vi "FGV - Path Registration.vi"(7 "FGV State":T1=enum."Register Path", 8 "error in (no error)":errorcluster, 10 "Path":path, 11 "Key":variant) -> (0 "error out":errorcluster, 1 "Key Already Included?":bool, 2 "Key Not Found?":bool, 3 "Path Out":path, 4 "Value Unchanged?":bool, 5 "All Paths":path[](array[path]))   [LabVIEW 2021, in "Path Utilities.lvlib"]
doc: "FGV for \"Path Registration\" VIs.\nNo error are generated inside this FGV."
uses:
  Path Utilities.lvlib
  TypeDefs/FGV State - Path Registration.ctl
  TypeDefs/FGV Data - Path Registration.ctl
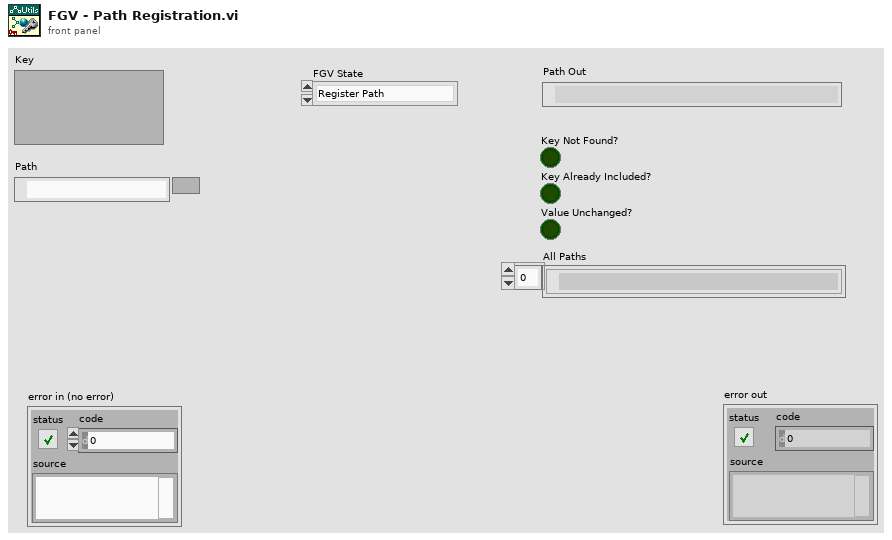
[diagram p1: front panel]
types:
  T1 = typedef "Path Utilities.lvlib/FGV State - Path Registration.ctl" = enum16{"Get Path", "List All Paths", "Register Path", "Unregister Path"}
  T2 = typedef "Path Utilities.lvlib/FGV Data - Path Registration.ctl" = cluster{"Path Map":map{variant, path}}
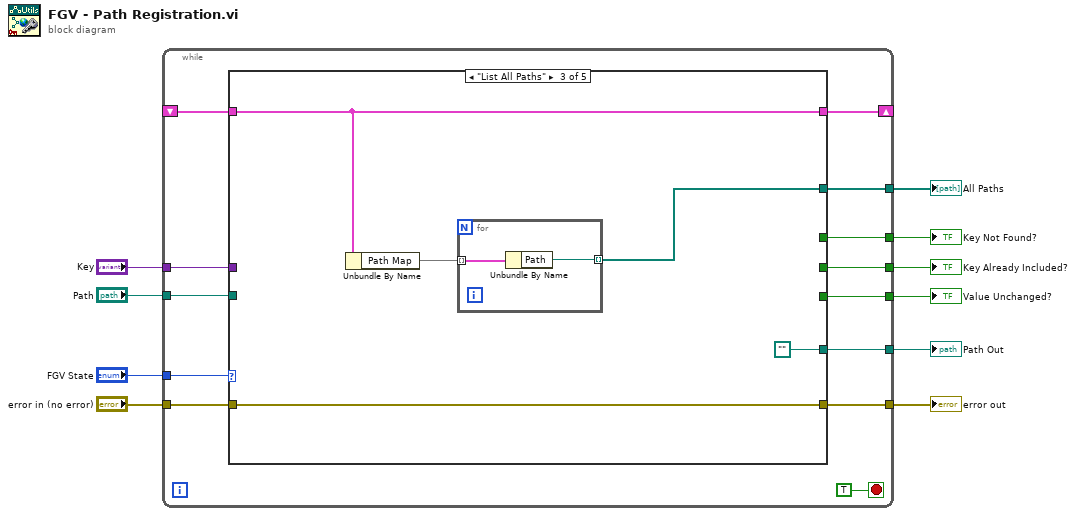
[diagram p0: block diagram]
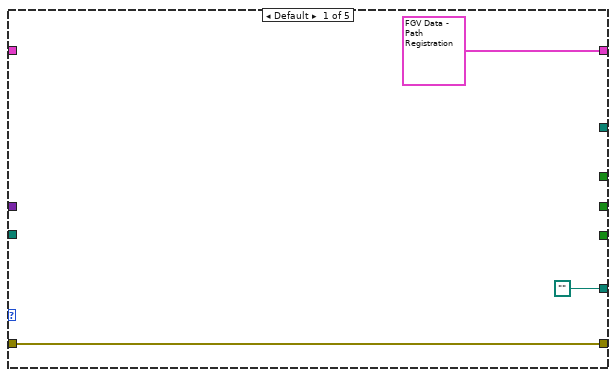
[diagram p2: hidden frame]
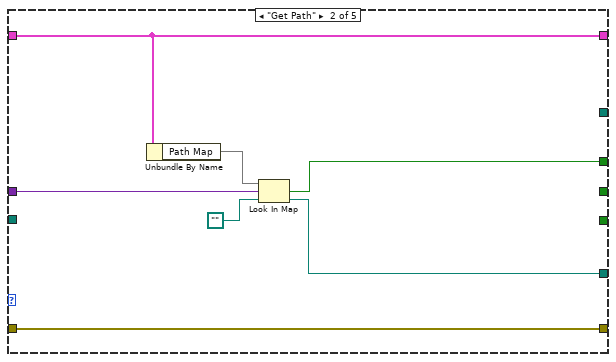
[diagram p3: hidden frame]
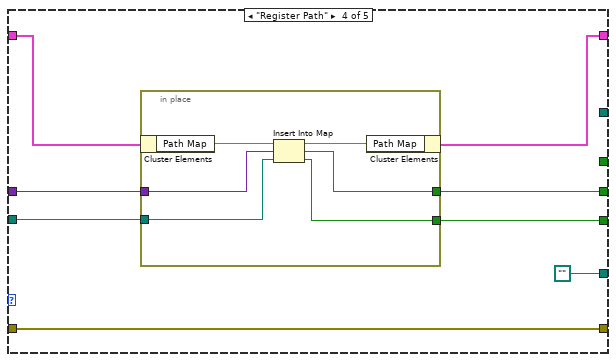
[diagram p4: hidden frame]
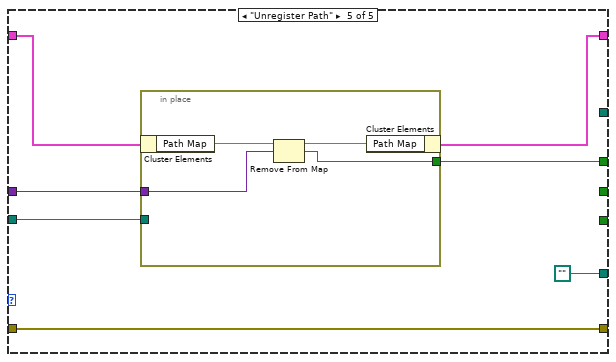
[diagram p5: hidden frame]
diagram:
  n1 = while {
    shift-right: [w19] -> _
    shift-left: _ -> [w17]
    tunnel: "FGV State" -> [w22]
    tunnel: "error in (no error)" -> [w21]
    tunnel: [w20] -> w9
    tunnel: "Path" -> [w18]
    tunnel: "Key" -> [w16]
    tunnel: [w15] -> w5
    tunnel: [w14] -> w4
    tunnel: [w13] -> w3
    tunnel: [w12] -> w2
    tunnel: [w11] -> w1
    stop <- TRUE stop-if-true
    n2 = case shown="\"List All Paths\"" w22 {
      tunnel: w21 -> [w26 w27 w35 w44 w57]
      tunnel: [w26 w27 w35 w44 w57] -> w20
      tunnel: [T2 {"Path Map"={}} ("FGV Data") w33 w38 w47 w60] -> w19
      tunnel: w18 -> [_ _ _ w45 w58]
      tunnel: w17 -> [_ w33 w38 w48 w61]
      tunnel: w16 -> [_ w32 _ w46 w59]
      tunnel: [_ _ _ w43 _] -> w15
      tunnel: [_ _ _ w42 _] -> w14
      tunnel: [path "" w29 path "" path "" path ""] -> w13
      tunnel: [_ w28 _ _ w56] -> w12
      tunnel: [_ _ w36 _ _] -> w11
      frame Default {
      }
      frame "Get Path" {
        n3 = Unbundle By Name(w33) -> ("Path Map"=w31:map{variant, path})
        n4 = Look In Map(map=w31, key=w32, default value=path "") -> (key not found?=w28:bool, value=w29:path)
      }
      frame "List All Paths" {
        n5 = Unbundle By Name(w38) -> ("Path Map"=w37:map{variant, path})
        n6 = for {
          tunnel: w37 -> [w40] mode=indexing
          tunnel: [w39] -> w36 mode=indexing
          n7 = Unbundle By Name(w40) -> ("Path"=w39:path)
        }
      }
      frame "Register Path" {
        n8 = in-place {
          in-place-border: w46 -> [w52]
          in-place-border: w45 -> [w51]
          in-place-border: [w50] -> w43
          in-place-border: [w49] -> w42
          n9 = in-place-cluster #1(w48) -> ("Path Map"=w54:map{variant, path})
          n10 = Insert Into Map(map in=w54, key=w52, value=w51) -> (map out=w53:map{variant, path}, key already included?=w50:bool, value unchanged?=w49:bool)
          n11 = in-place-cluster #1("Path Map"=w53) -> (w47:T2)
        }
      }
      frame "Unregister Path" {
        n12 = in-place {
          in-place-border: w59 -> [w65]
          in-place-border: w58 -> [_]
          in-place-border: [w62] -> w56
          n13 = in-place-cluster #2(w61) -> ("Path Map"=w64:map{variant, path})
          n14 = Remove From Map(10:w65, 11:w64) -> (2:w62:bool, 3:w63:map{variant, path})  [unwired: 1 out]
          n15 = in-place-cluster #2("Path Map"=w63) -> (w60:T2)
        }
      }
    }
  }
  "error out" <- w9
  "Path Out" <- w3
  "Key Already Included?" <- w5
  "Value Unchanged?" <- w4
  "Key Not Found?" <- w2
  "All Paths" <- w1
